vi "Request Motors with Encoders State.vi"(8 "error in (no error)":errorcluster, 9 "Requestor Queue":refnum<class "Message Enqueuer.lvclass">, 10 "Current State Msg":refnum<class "Current State Msg.lvclass">, 11 "Motors with Encoders in":refnum<class "Motors with Encoders.lvclass">) -> (0 "error out":errorcluster, 3 "Motors with Encoders out":refnum<class "Motors with Encoders.lvclass">)   [LabVIEW 2014, in "Motors with Encoders.lvlib" / "Motors with Encoders.lvclass"]
uses:
  Motors with Encoders.lvclass
  Motors with Encoders Messages/Current State Msg/Current State Msg.lvclass
  <vilib>/ActorFramework/Message Enqueuer/Message Enqueuer.lvclass
  Motors with Encoders.lvclass/Motors with Encoders.ctl
  Motors with Encoders Messages/Current State Msg/Current State Msg.lvclass/Current State Msg.ctl
  <vilib>/ActorFramework/Message Enqueuer/Message Enqueuer.lvclass/Message Enqueuer.ctl
  <vilib>/ActorFramework/Message Enqueuer/Enqueue.vi
  <vilib>/ActorFramework/Message Priority Queue/Priority Enqueue.vi
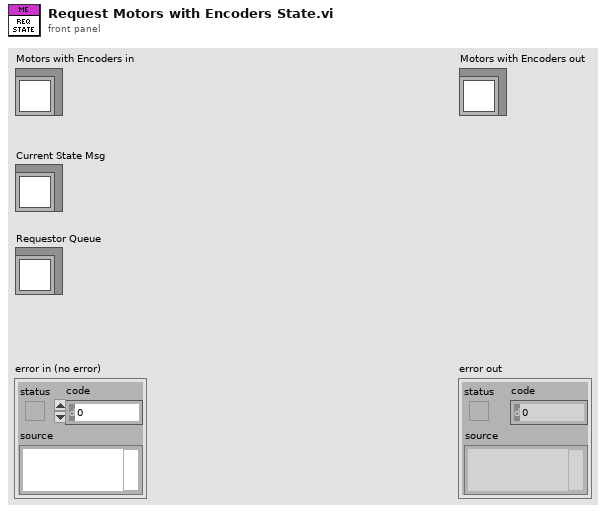
[diagram p1: front panel]
types:
  T1 = typedef "Motors with Encoders.lvlib/Motors with Encoders.lvclass/Motors with Encoders State.ctl" = cluster{"Forward Switch":bool, "Reverse Switch":bool, "Measured RPM":dbl, "Distance (in)":dbl, "Setpoint RPM":dbl, "Encoder Count":i64, "Home Count":i64, "Config":T2}
  T2 = typedef "Motors with Encoders.lvlib/Motors with Encoders.lvclass/Motors with Encoders Config.ctl" = cluster{"Counts  Per Revolution":u32, "Invert Encoder Direction":bool, "Diameter of Revolution":dbl, "Max RPM":dbl, "Encoder Control":bool}
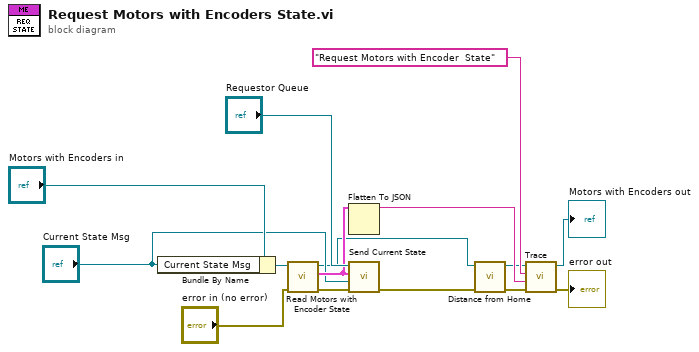
[diagram p0: block diagram]
diagram:
  n1 = Bundle By Name(cluster="Motors with Encoders in", "Current State Msg"="Current State Msg") -> (w14:refnum<class "Motors with Encoders.lvclass">)
  n2 = call-dynamic "Read Motors with Encoder State.vi"("error in (no error)"="error in (no error)", "Motors with Encoders in"=w14) -> ("error out"=w3:errorcluster, "Motors with Encoder State"=w7:T1, "Motors with Encoders out"=w5:refnum<class "Motors with Encoders.lvclass">)  [unwired: 7 in]
  n3 = Flatten To JSON(anything=w7) -> (JSON string=w9:string)  [unwired: 2 in, 1 out]
  n4 = call "Send Current State.vi"("error in (no error)"=w3, "Motors with Encoders.lvlib:Current State Msg.lvclass"="Current State Msg", "Motors with Encoder State"=w7, "Message Enqueuer"="Requestor Queue") -> ("error out"=w2:errorcluster)  [unwired: 6 in, 1 out]
  n5 = call-dynamic "Distance from Home.vi"("error in (no error)"=w2, "Motors with Encoders in"=w5) -> ("error out"=w1:errorcluster, "Motors with Encoders out"=w4:refnum<class "Motors with Encoders.lvclass">)  [unwired: 8 in]
  n6 = call-dynamic "Trace.vi"("error in (no error)"=w1, "System Message"=w9, "System Action"="Request Motors with Encoder  State", "System Actor in"=w4) -> ("error out"=→"error out":errorcluster, "System Actor out"=→"Motors with Encoders out":refnum<class "Motors with Encoders.lvclass">)  [unwired: 6 in]
